vi "asdasd.vi"() -> ()   [LabVIEW 2018]
uses:
  <vilib>/userdefined/High Color/IMAQdx.ctl
  <vilib>/vision/driver/NI_Vision_Acquisition_Software.lvlib
panel:
  out "Frame Rate":dbl(knob) scale=0.0..100.0
  out "Image":T1(plugin-control)
  out "큐의 원소 개수":i32(slide) scale=0.0..50.0
  in  "정지 버튼":bool
  out "Buffer Number Out":u32
  in  "Session In":T2
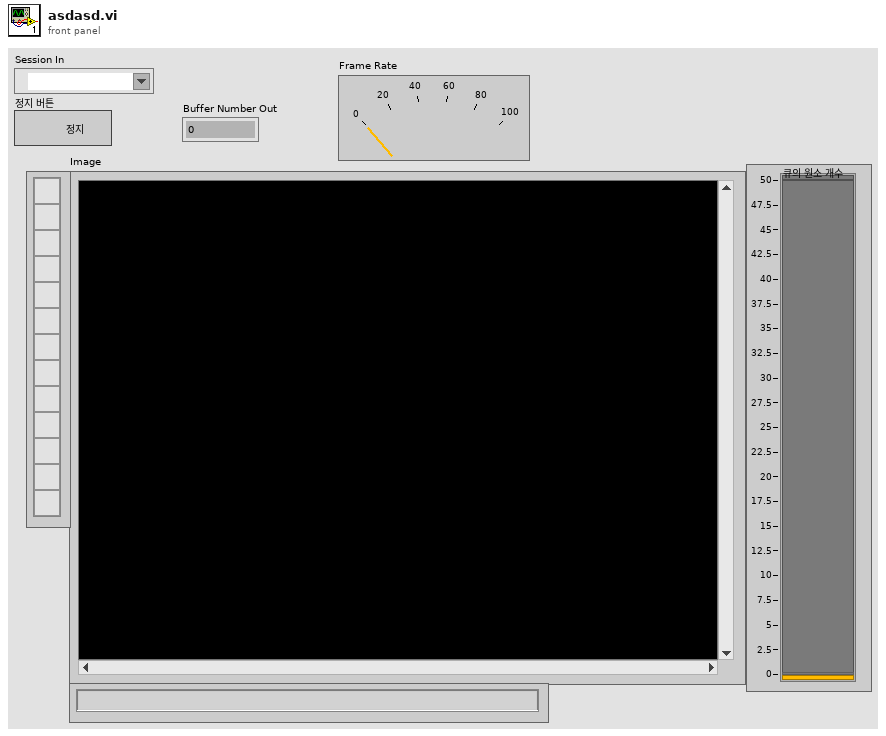
[diagram p1: front panel]
types:
  T1 = typedef "IMAQ Image.ctl" = refnum<image>
  T2 = typedef "IMAQdx.ctl" = refnum<k21>
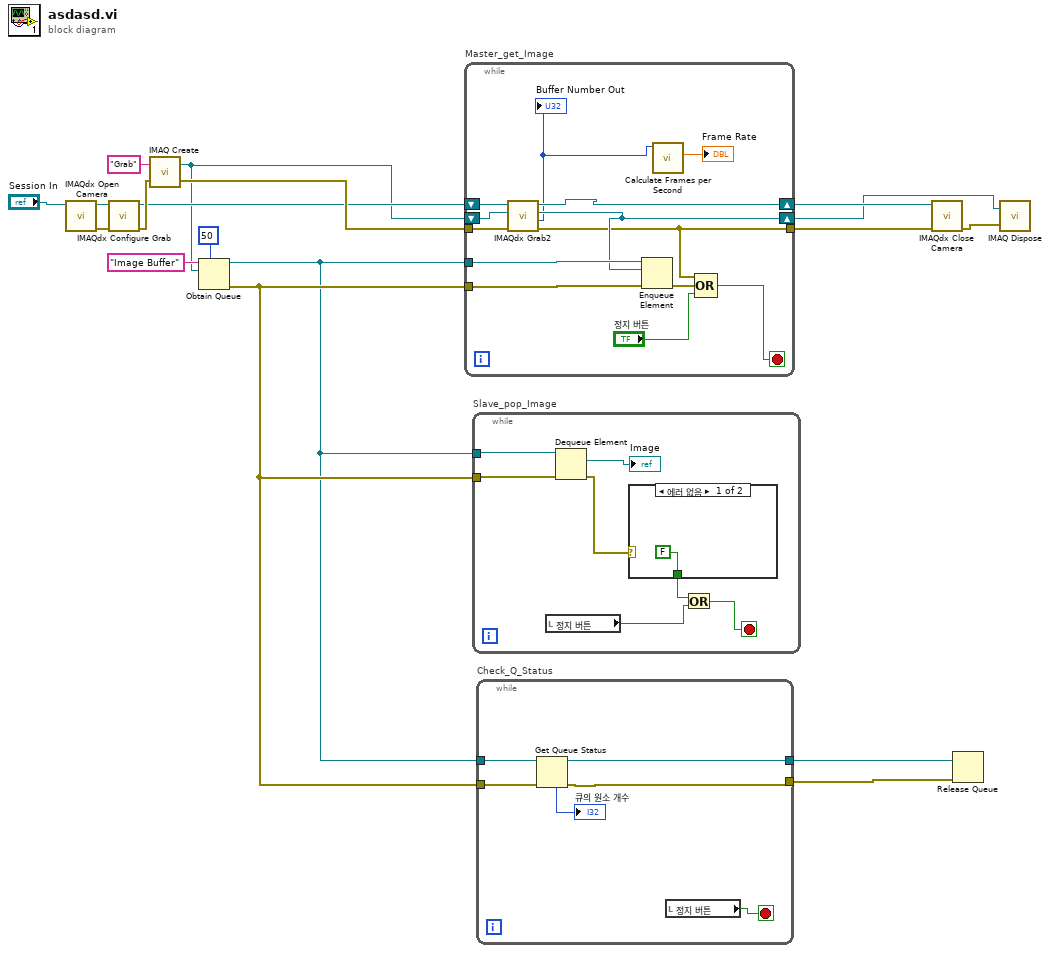
[diagram p0: block diagram]
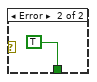
[diagram p2: hidden frame]
diagram:
  n1 = call <vilib>:"IMAQdx Open Camera.vi"("Session In"="Session In") -> ("error out"=w17:errorcluster, "Session Out"=w18:T2)  [unwired: 9 in]
  n2 = call <vilib>:"IMAQdx Configure Grab.vi"("error in"=w17, "Session In"=w18) -> ("error out"=w16:errorcluster, "Session Out"=w14:T2)  [unwired: 8 in]
  n3 = call "IMAQ Create"("Image Name"="Grab", "error in (no error)"=w16) -> ("New Image"=w5:T1, "error out"=w15:errorcluster)  [unwired: 3 in]
  n4 = Obtain Queue(max queue size (-1, unlimited)=50 ("최대 큐 크기(-1,제한없음)"), name (unnamed)="Image Buffer" ("이름(이름없음)"), element data type=w5) -> (queue out=w3:refnum<queue>, error out=w4:errorcluster)  [unwired: 2 in, 1 out]
  n5 = while "Master_get_Image" {
    tunnel: w15 -> [w31]
    tunnel: [w21] -> w10
    tunnel: w3 -> [w28]
    tunnel: w4 -> [w27]
    shift-right: [w23] -> w11
    shift-left: w14 -> [w30]
    shift-right: [w22] -> w7
    shift-left: w5 -> [w29]
    stop <- w24 stop-if-true
    n6 = call <vilib>:"IMAQdx Grab2.vi"("error in"=w31, "Image In"=w29, "Session In"=w30) -> ("error out"=w21:errorcluster, "Buffer Number Out"=w19:u32, "Image Out"=w22:T1, "Session Out"=w23:T2)  [unwired: 5 in]
    "Buffer Number Out" <- w19
    n7 = Enqueue Element(queue=w28, element=w22, error in (no error)=w27) -> (error out=w26:errorcluster)  [unwired: 1 in, 2 out]
    n8 = call <vilib>:"Calculate Frames per Second.vi"("Buffer Number"=w19) -> ("Processed Frames/s"=→"Frame Rate":dbl)  [unwired: 8 in, 2 out]
    n9 = Compound Arithmetic op=OR(w21, w26, "정지 버튼") -> (w24:bool)
  }
  n10 = while "Slave_pop_Image" {
    tunnel: w4 -> [w36]
    tunnel: w3 -> [w37]
    stop <- w32 stop-if-true
    n11 = local read "정지 버튼"() -> (w33:bool)
    n12 = Dequeue Element(queue=w37, error in (no error)=w36) -> (element=→"Image":T1, error out=w35:errorcluster)  [unwired: 1 in, 2 out]
    n13 = case shown="에러 없음" w35 {
      tunnel: [FALSE TRUE] -> w34
      frame No Error {
      }
      frame Error {
      }
    }
    n14 = Or(x=w34, y=w33) -> (x .or. y?=w32:bool)
  }
  n15 = while "Check_Q_Status" {
    tunnel: w4 -> [w46]
    tunnel: w3 -> [w45]
    tunnel: [w43] -> w2
    tunnel: [w42] -> w1
    stop <- w41 stop-if-true
    n16 = Get Queue Status(queue=w45, error in (no error)=w46) -> (queue out=w42:refnum<queue>, error out=w43:errorcluster, # elements in queue=→"큐의 원소 개수":i32)  [unwired: 1 in, 5 out]
    n17 = local read "정지 버튼"() -> (w41:bool)
  }
  n18 = call <vilib>:"IMAQdx Close Camera.vi"("error in"=w10, "Session In"=w11) -> ("error out"=w9:errorcluster)  [unwired: 9 in]
  n19 = Release Queue(queue=w1, error in (no error)=w2) -> ()  [unwired: 1 in, 3 out]
  n20 = call "IMAQ Dispose"("Image"=w7, "error in (no error)"=w9) -> ()  [unwired: 4 in, 1 out]
